vi "AlliGator Load ROI v3.vi"(7 "File Path":path, 8 "Error In":errorcluster, 9 "Destination Image (Source Image)":string="Source Image", 10 "Dialog (T)":bool=TRUE, 11 "Source Image Refnum":T3) -> (0 "Error Out":errorcluster, 1 "Current ROI":i32, 2 "Updated ROIs":T1[](array[typedef]) {"ROI Descriptor"."Contours"."Type" items=["No Selection", "Point", "Line", "Rectangle", "Oval", "Polygon", "Freehand Region", "Annulus", "Unused2", "Unused3", "Broken Line", "Freehand Line", "Rotated Rectangle"]}, 3 "Message":string, 4 "Phasor Plot Image":bool, 5 "# ROIs Loaded":i32, 6 "Time (s)":dbl)   [LabVIEW 2021, in "AlliGator ROIs.lvlib"]
doc: "When invoked from a context menu, used Dialog for file selection: the Dialog flag should be set to True (default) and the Destination Image string is ignored.\n\nWhen invoked from a drag & drop event, the Dialog flag should be set to False and the Destination Image (Source Image or Phasor Plot Image) should be provided."
uses:
  AlliGator ROIs.lvlib
  Image/Image Control Refnum.ctl
  Image/Named ROI Description.ctl
  Globals, Variables, Constants/AlliGator Refnums List.ctl
  Globals, Variables, Constants/AlliGator Variables List.ctl
  Image/ROI XML Format.ctl
  Image/Image Control ROI Description.ctl
  Image/Image Control Multiple ROIs Description.ctl
  Image/Image Control ROI Description v2.ctl
  Image/Image Control Multiple ROIs Description v2.ctl
  AlliGator ROI Manager Actions.ctl
  8ad5fe3a-6877-4cbc-8fef-4c072b65eab6.vi
  454e6171-cdfd-4cb8-a5e3-eaa046060a80.vi
  Variant/Variant to Data/Variant to I32.vi
  <vilib>/JDP Science/JSONtext/JSON text to Variant.vi
  <vilib>/Utility/error.llb/Error Cluster From Error Code.vi
  <vilib>/JDP Science/JSONtext/LVClass Serializer/JSONtext LVClass Serializer.lvclass
  <vilib>/ErrorRing/Error Ring.xnode
  Image/Image.lvlib
  Files/Files.lvlib
  Error/Error.lvlib
  Globals, Variables, Constants/AlliGator Globals, Variables & Constants.lvlib
  Variant/Variant to Data/Variant to Data.lvlib
  Time/Time.lvlib
  Sound/Sound.lvlib
panel:
  # "see the AlliGator License on the block diagram (Ctrl+E or Window:Show Block Diagram)"
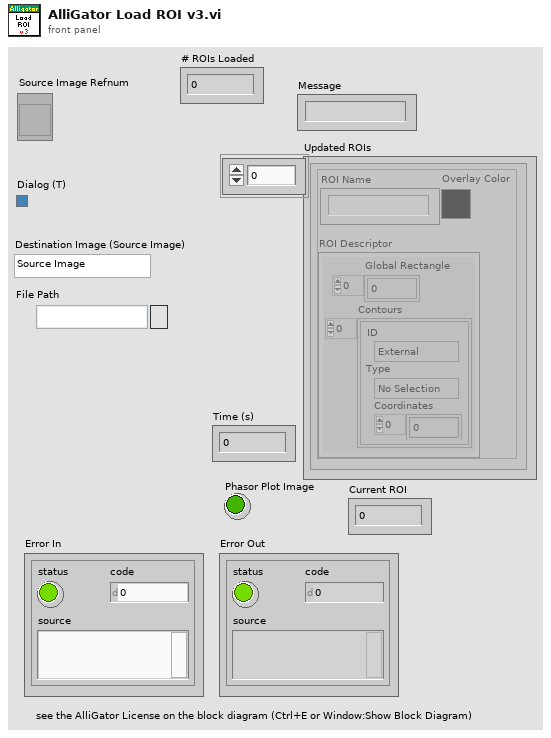
[diagram p1: front panel]
types:
  T1 = typedef "Image.lvlib/Named ROI Description.ctl" = cluster{"ROI Descriptor":T2, "ROI Name":string, "Overlay Color":u32}
  T2 = typedef "ROI Descriptor" = cluster{"Global Rectangle":i32[], "Contours":cluster{"ID":enum32{"External", "Internal"}, "Type":u32, "Coordinates":i32[]}[]}
  T3 = typedef "Image.lvlib/Image Control Refnum.ctl" = refnum<vi>
  T4 = typedef "AlliGator Globals, Variables & Constants.lvlib/AlliGator Refnums List.ctl" = enum16{"---------- AlliGator Controls ----------", "AlliGator Tab Control Refnum", "---------- AlliGator Indicators ----------", "Source Image Display Refnum", "Phasor Plot Display Refnum", "Decay Fit Parameter Map Refnum", "---------- AlliGator VIs ----------", "AlliGator Refnum", "AlliGator Settings Refnum", "AlliGator Launcher Refnum"}
  T5 = typedef "AlliGator Globals, Variables & Constants.lvlib/AlliGator Variables List.ctl" = enum16{"---- GUI ----", "GUI:Initialization Status", "GUI:State Indicators Refnum", "GUI:Original AlliGator Menu Items", "GUI:Current Action Loop State", "GUI:Script in progress", "GUI:Playback", "GUI:Loop Playback", "GUI:Search ROI Used", "GUI:Search ROI", "Decay Graph Max Legend Size", "Intensity Graph Max Legend Size", "Decay Statistics Graph Max Legend Size", "Phasor Graph Max Legend Size", "Phasor Ratio Graph Max Legend Size", "Lifetime Graph Max Legend Size", "---- Files ----", "Files:Export Dataset Frames as Individual Files", "Files:Show Batch Export Help Balloons", "Files:Frames in Dataset", "Files:ptu File Frame Start Indices", "Files:Current Frame in Dataset", "Files:Current Frame Timestamp", "Files:Dataset Loaded", "Files:Dataset Metadata", "Files:Dataset Channel", "Files:Dataset Data Description", "Files:Background Dataset Metadata", "Files:Background Dataset Channel", "Files:Background Dataset Data Description", "Files:Background File Subtraction", "Files:Background File Path", "Files:Background File Pile-up Correction", "Files:Background File Pixel Well Capacity", "Files:Background File Scaling Factor", "Files:Current Dataset Load Settings", "Files:Dataset Path", "Files:ICCD-specific Information", "Files:Macrotime Gate Separation", "------ Python Plugins ------", "Python Plugins:Information", "Python Plugins:Python Session", "Python Plugins:Valid Python Session?", "---- Source Image ----", "Source Image:ROIs", "Source Image:Current ROI", "Source Image:ROI Event Refnum", "X_Source Image:Display Range", "X_Source Image:Palette Information", "X_Source Image:Type of Displayed Image", "X_Time Gate Slider", "Source Image:Palette List", "Source Image:Scale", "Source Image:ROI Overlay Color", "Source Image:Overlay to Erase", "Source Image:Is Displayed Image Accumulated", "Source Image:White Light Image Modified", "Source Image:Mask Image Modified", "---- Image Profile Window ----", "Image Profile:Window Event Refnum", "Image Profile:IntensityType", "Image Profile:Intensity Average Type", "Image Profile:Intensity-weighted SDV", "Image Profile:Box Profile Type", "Image Profile:Window Open", "Image Profile:Plotted Fit Parameter", "------ Phasor Graph -------", "Phasor Graph:Show Line", "---- Phasor Plot ---", "Phasor Plot:Parameters Changed", "Phasor Plot:FLI Dataset Modified since last Calculation", "Phasor Harmonics Data", "Selected Phasor Harmonics", "Phasor Harmonic Manager Event Refnum", "Phasor Plot:ROIs", "Phasor Plot:Current ROI", "Phasor Plot:ROI Event Refnum", "Phasor Plot:Image Reference Points", "Phasor Plot:Computed", "Phasor Plot:Palette Information", "Phasor Plot:Palette List", "Phasor Plot:Phasor Ratio Palette Information", "Phasor Plot:Phasor Ratio Palette List", "Phasor Plot:Image Scale", "Phasor Plot:Image Overlay to Erase", "Phasor Plot:Image Elements to Update", "Phasor Plot:Current Calculation Parameters", "Phasor Plot:Current Calibration Options", "Phasor Plot:Reset Cumulated Phasor Plot", "Phasor Plot:Reference 1", "Phasor Plot:Lifetime Reference 1", "Phasor Plot:Reference 1 Frequency", "Phasor Plot:Reference 2", "Phasor Plot:Lifetime Reference 2", "Phasor Plot:Reference 2 Frequency", "---- Decay Analysis ----", "Number of Selected Decays to Fit", "LS Fit Results", "LAR Fit Results", "BS Fit Results", "Last Decay Max - Min", "Best Fit Parameters", "Best Fit Parameter Names", "Actual Size X", "Actual Size Y", "Binning X", "Binning Y", "Actual # Gates", "Dataset Number", "Gates to...", "Gates Skipped", "Gates to keep", "Gate Step", "Gate Separation", "Reversed Gates", "Pile-up Correction", "Pixel Well Capacity", "Background Subtracted", "Background Subtraction Method", "Background Definition Range", "Background File (deprecated)", "Number of Dataset Accumulated", "Array of Accumulated Dataset Paths", "Do Averaged Datasets", "Destination File Path", "Process Plot Target", "Use 1/D as Phasor Frequency", "---- Decay Fit Parameter Map -----", "Decay Fit Parameter Map:Palette Information", "Decay Fit Parameter Map:Palette List", "Decay Fit Parameter Map:X Resolution", "Decay Fit Parameter Map:Y Resolution", "---- Parameter Map ----", "Parameter Map:Palette Information", "Parameter Map:Palette List", "------- Local Decay Window ---------", "Local Decay Graph Window:Event Refnum", "Local Decay Graph Window:Use normalized IRF for convolution", "----- Miscellaneous ----", "Misc:Skippable Dialog Windows Status"}
  T6 = typedef "Image.lvlib/ROI XML Format.ctl" = enum16{"Single ROI v1", "Multiple ROIs v1", "Single ROI v2", "Multiple ROIs v2", "Single ROI v3", "Multiple ROIs v3", "Exit"}
  T7 = typedef "Image.lvlib/Image Control ROI Description.ctl" = cluster{"Image Control Label":string, "ROI Descriptor":T2}
  T8 = typedef "Image.lvlib/Image Control Multiple ROIs Description.ctl" = cluster{"Image Control Label":string, "ROI Descriptors":T2[]}
  T9 = typedef "Image.lvlib/Image Control ROI Description v2.ctl" = cluster{"Image Control Label":string, "Named ROI Description":T1}
  T10 = typedef "Image.lvlib/Image Control Multiple ROIs Description v2.ctl" = cluster{"Image Control Label":string, "Named ROI Descriptions":T1[]}
  T11 = typedef "AlliGator ROIs.lvlib/AlliGator ROI Manager Actions.ctl" = enum16{"Undefined", "Delete Current ROI", "Delete All Unselected ROIs", "Delete Multiple ROIs", "Delete All ROIs", "Swap ROIs", "Insert ROI", "Update Current ROI Descriptor", "Rename Current ROI", "Store New ROI", "Store Multiple ROIs", "Select Next ROI", "Select Previous ROI", "Find Selected ROI", "Show All ROIs", "Update ROI Manager Window", "Merge All ROIs", "Unmerge ROI", "Set Selected ROI by ID"}
  T12 = typedef "AlliGator ROIs.lvlib/AlliGator Image ROI Event refnum.ctl" = refnum<user-event>
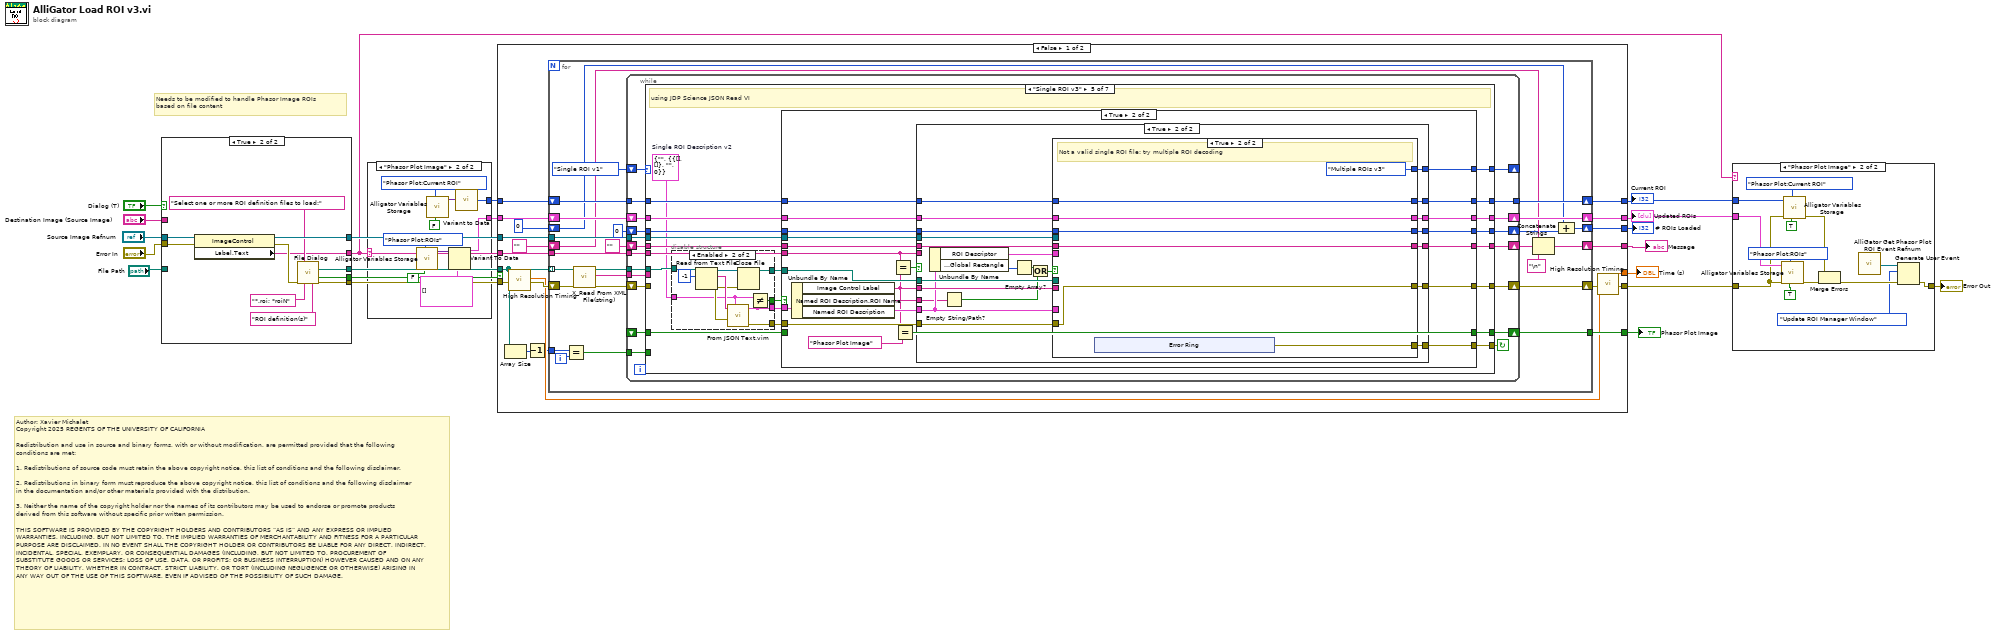
[diagram p0: block diagram]
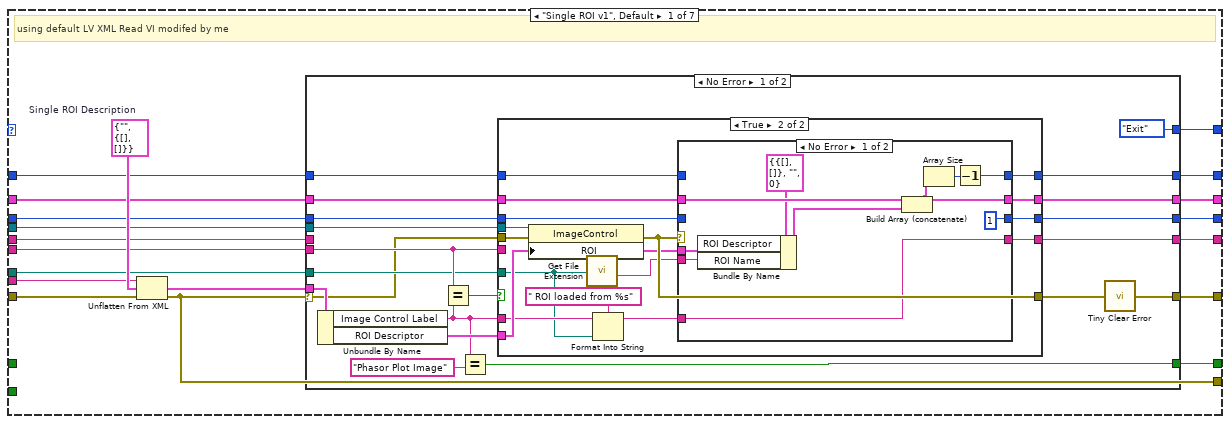
[diagram p2: hidden frame]
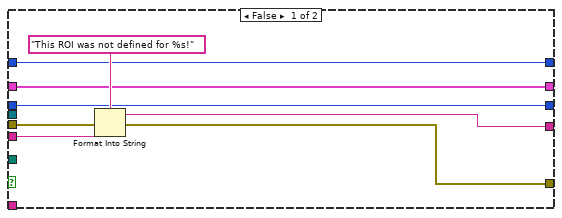
[diagram p3: hidden frame]
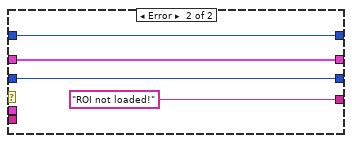
[diagram p4: hidden frame]
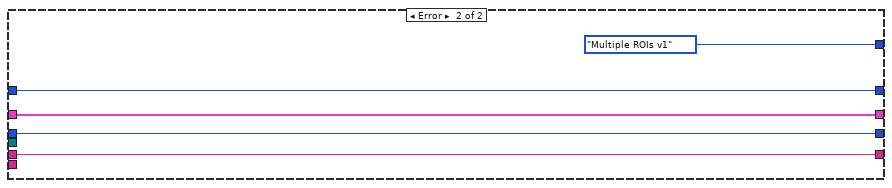
[diagram p5: hidden frame]
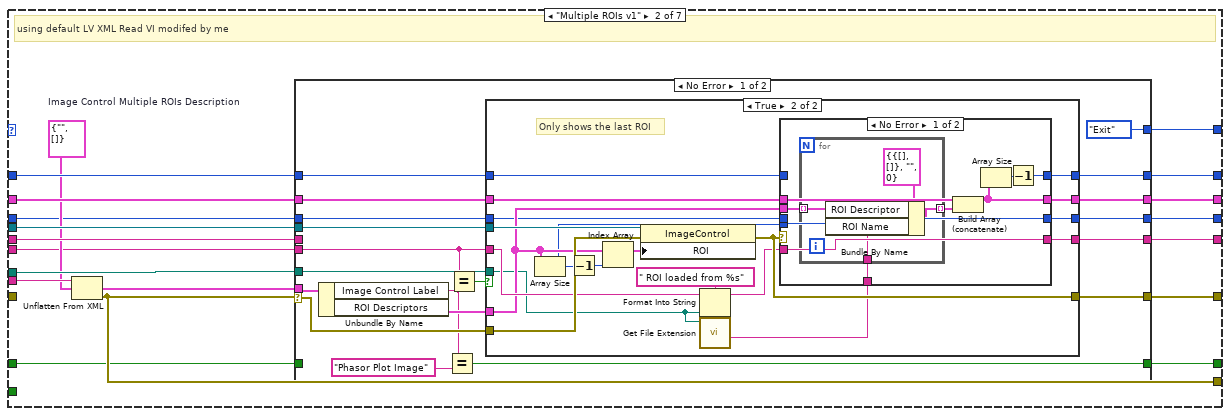
[diagram p6: hidden frame]
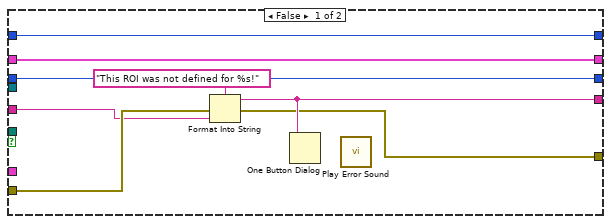
[diagram p7: hidden frame]
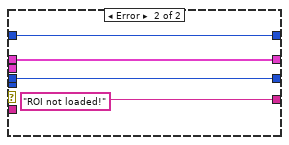
[diagram p8: hidden frame]
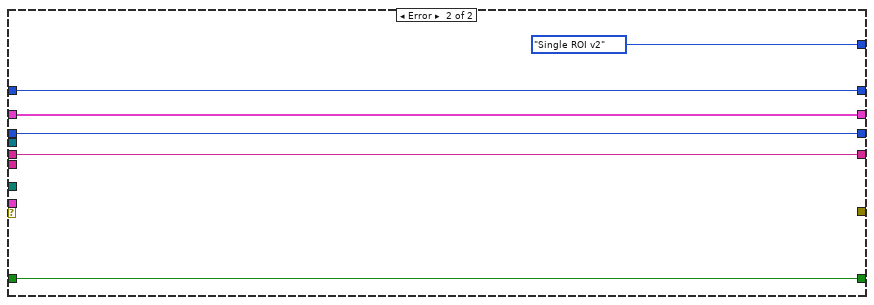
[diagram p9: hidden frame]
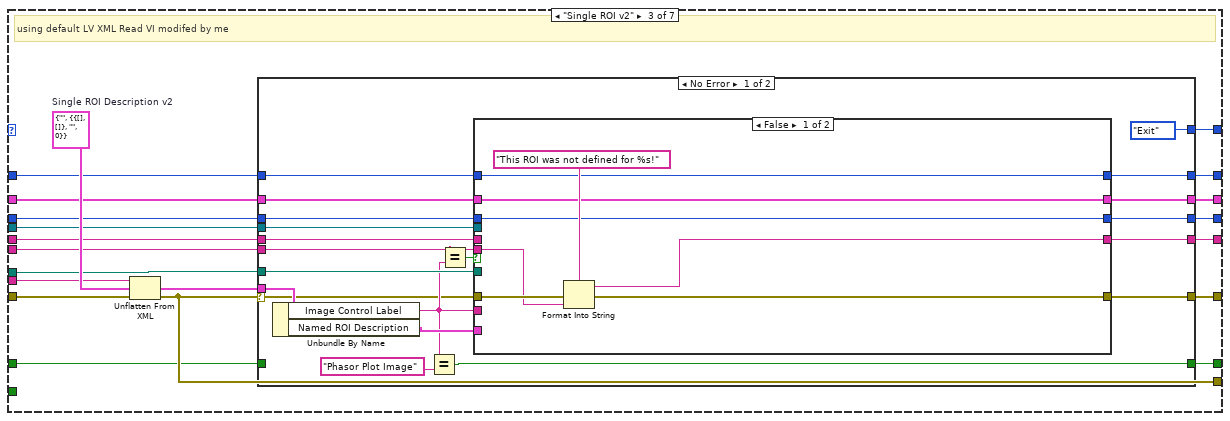
[diagram p10: hidden frame]
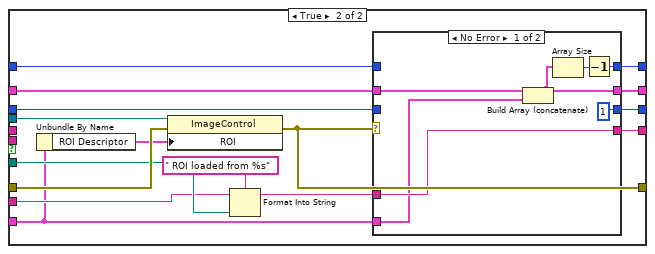
[diagram p11: hidden frame]
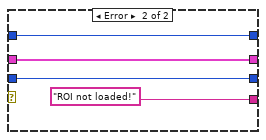
[diagram p12: hidden frame]
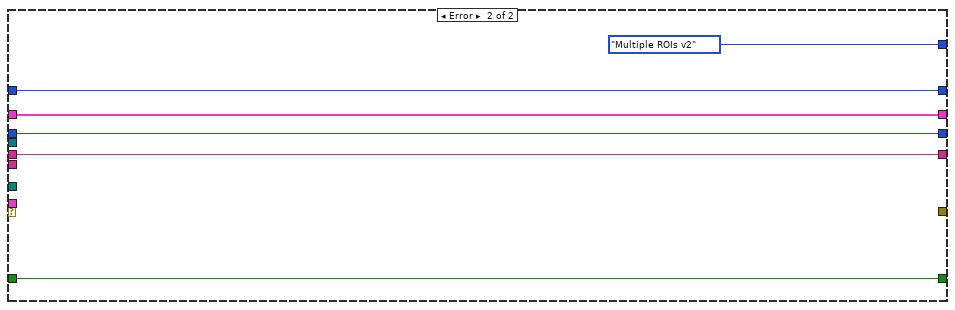
[diagram p13: hidden frame]
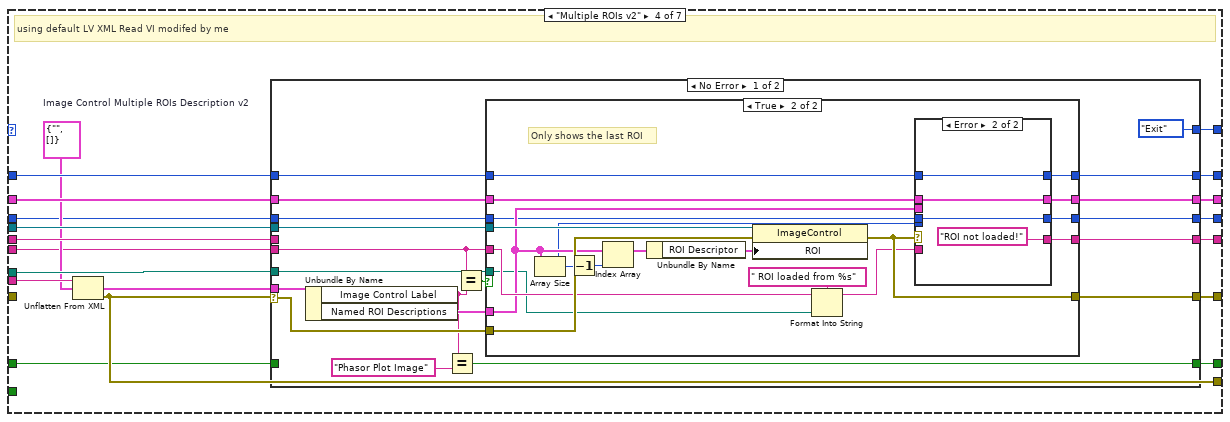
[diagram p14: hidden frame]
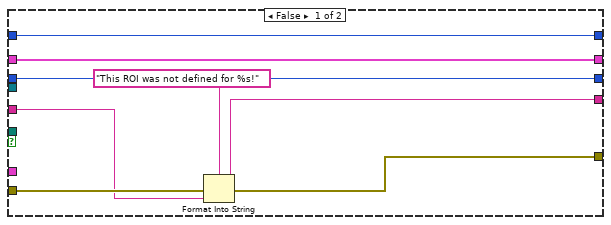
[diagram p15: hidden frame]
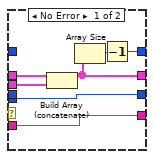
[diagram p16: hidden frame]
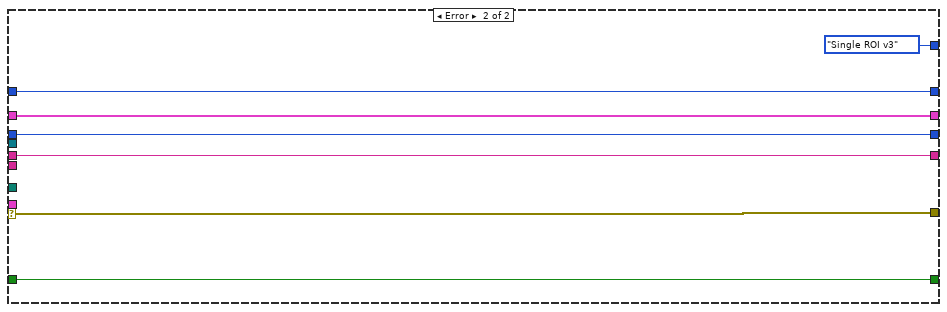
[diagram p17: hidden frame]
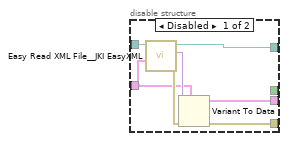
[diagram p18: hidden frame]
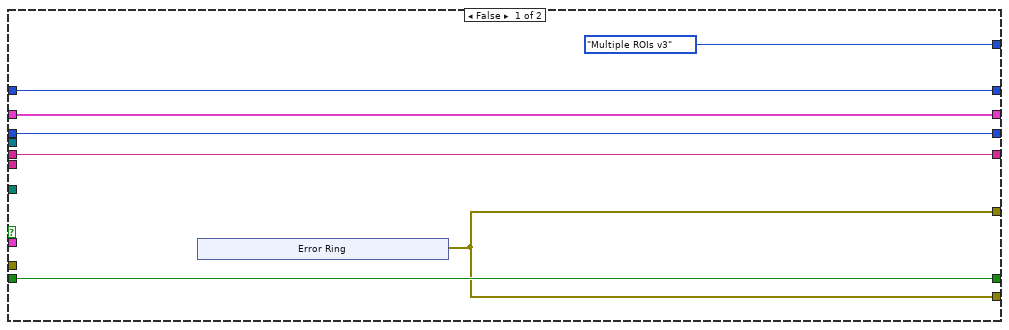
[diagram p19: hidden frame]
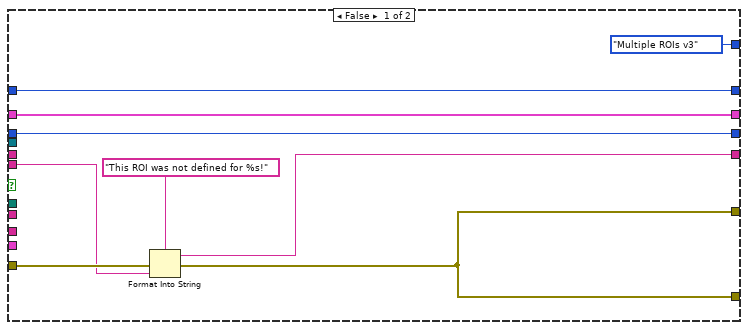
[diagram p20: hidden frame]
diagram:
  # "Author: Xavier Michalet\nCopyright 2025 REGENTS OF THE UNIVERSITY OF CALIFORNIA\n\nRedistribution and use in source and binary forms, with or without modification, are permitted provided that the following conditions are met:\n\n1. Redistributions of source code must retain the above copyright notice, this list of conditions and the following disclaimer.\n\n2. Redistributions in binary form must reproduce the above copyright notice, this list of conditions and the following disclaimer in the documentation and/or other materials provided with the distribution.\n\n3. Neither the name of the copyright holder nor the names of its contributors may be used to endorse or promote products derived from this software without specific prior written permission.\n\nTHIS SOFTWARE IS PROVIDED BY THE COPYRIGHT HOLDERS AND CONTRIBUTORS “AS IS” AND ANY EXPRESS OR IMPLIED WARRANTIES, INCLUDING, BUT NOT LIMITED TO, THE IMPLIED WARRANTIES OF MERCHANTABILITY AND FITNESS FOR A PARTICULAR PURPOSE ARE DISCLAIMED. IN NO EVENT SHALL THE COPYRIGHT HOLDER OR CONTRIBUTORS BE LIABLE FOR ANY DIRECT, INDIRECT, INCIDENTAL, SPECIAL, EXEMPLARY, OR CONSEQUENTIAL DAMAGES (INCLUDING, BUT NOT LIMITED TO, PROCUREMENT OF SUBSTITUTE GOODS OR SERVICES; LOSS OF USE, DATA, OR PROFITS; OR BUSINESS INTERRUPTION) HOWEVER CAUSED AND ON ANY THEORY OF LIABILITY, WHETHER IN CONTRACT, STRICT LIABILITY, OR TORT (INCLUDING NEGLIGENCE OR OTHERWISE) ARISING IN ANY WAY OUT OF THE USE OF THIS SOFTWARE, EVEN IF ADVISED OF THE POSSIBILITY OF SUCH DAMAGE."
  # "Needs to be modified to handle Phasor Image ROIs\nbased on file content"
  n1 = case shown="True" "Dialog (T)" {
    tunnel: "Source Image Refnum" -> [_ w46]
    tunnel: [w22 w45] -> w19
    tunnel: "Error In" -> [w21 w44]
    tunnel: [w21 w42] -> w16
    tunnel: [w24 w38] -> w15
    tunnel: [_ w37] -> w13
    tunnel: [w23 w36] -> w8
    tunnel: "Destination Image (Source Image)" -> [w23 _]
    tunnel: "File Path" -> [w25 _]
    frame False {
      # "Drag & Drop event"
      n2 = case shown="\"Phasor Plot Image\"" w23 {
        tunnel: [w27 w32] -> w22
        frame "Source Image", Default {
          n3 = call "AlliGator Refnums Storage.vi"("AlliGator Refnum List"=AlliGator_Refnums_List."Source Image Display Refnum") -> ("Error Out"=w29:errorcluster, "Data out"=w30:variant)  [unwired: 9 in]
          n4 = Variant To Data(error in=w29, type=refnum<vi> refnum ("Image Source Refnum"), Variant=w30) -> (data=w27:refnum<vi>)  [unwired: 1 out]
        }
        frame "Phasor Plot Image" {
          n5 = call "AlliGator Refnums Storage.vi"("AlliGator Refnum List"=AlliGator_Refnums_List."Phasor Plot Display Refnum") -> ("Error Out"=w34:errorcluster, "Data out"=w35:variant)  [unwired: 9 in]
          n6 = Variant To Data(error in=w34, type=refnum<vi> refnum ("Image Source Refnum"), Variant=w35) -> (data=w32:refnum<vi>)  [unwired: 1 out]
        }
      }
      n7 = Build Array(w25) -> (w24:path[])
    }
    frame True {
      n8 = property class="ImageControl"(reference=w46, error in=w44) -> (reference out=w45:T3, error out=w43:errorcluster, "Label.Text"=w36:string)
      n9 = call "File Dialog"("prompt"="Select one or more ROI definition files to load:", "error in"=w43, "pattern (all files)"="*.roi; *roiN", "pattern label"="ROI definition(s)") -> ("selected paths"=w38:path[], "cancelled"=w37:bool, "error out"=w42:errorcluster)  [unwired: 8 in, 1 out]
    }
  }
  n10 = case shown="\"Phasor Plot Image\"" w8 {
    tunnel: [w53 w63] -> w12
    tunnel: [w47 w57] -> w11
    frame "Source Image", Default {
      n11 = call "Alligator Variables Storage.vi"("Get(F)/Set"=FALSE, "AlliGator Variable"=AlliGator_Variables_List."Source Image:ROIs" ("Alligator Variable")) -> ("Error Out"=w49:errorcluster, "Data out"=w50:variant)  [unwired: 7 in, 1 out]
      n12 = call "Alligator Variables Storage.vi"("Get(F)/Set"=FALSE, "AlliGator Variable"=AlliGator_Variables_List."Source Image:Current ROI" ("Alligator Variable")) -> ("Data out"=w54:variant)  [unwired: 7 in, 2 out]
      n13 = Variant To Data(error in=w49, type=T1[] [] ("Existing ROIs"), Variant=w50) -> (data=w47:T1[])  [unwired: 1 out]
      n14 = call-poly "Variant to Data.vi"("Variant"=w54) -> ("Value"=w53:i32)  [unwired: 8 in]
    }
    frame "Phasor Plot Image" {
      n15 = call "Alligator Variables Storage.vi"("Get(F)/Set"=FALSE, "AlliGator Variable"=AlliGator_Variables_List."Phasor Plot:ROIs" ("Alligator Variable")) -> ("Error Out"=w59:errorcluster, "Data out"=w60:variant)  [unwired: 7 in, 1 out]
      n16 = call "Alligator Variables Storage.vi"("Get(F)/Set"=FALSE, "AlliGator Variable"=AlliGator_Variables_List."Phasor Plot:Current ROI" ("Alligator Variable")) -> ("Data out"=w64:variant)  [unwired: 7 in, 2 out]
      n17 = Variant To Data(error in=w59, type=T1[] [] ("Existing ROIs"), Variant=w60) -> (data=w57:T1[])  [unwired: 1 out]
      n18 = call-poly "Variant to Data.vi"("Variant"=w64) -> ("Value"=w63:i32)  [unwired: 8 in]
    }
  }
  n19 = case shown="False" w13 {
    tunnel: w8 -> [w86 _]
    tunnel: w19 -> [w85 _]
    tunnel: w11 -> [w84 w728]
    tunnel: [w83 w728] -> w9
    tunnel: [w72 w729] -> w1
    tunnel: w12 -> [w81 _]
    tunnel: [w80 -1 ("Current ROI")] -> w10
    tunnel: [w79 _] -> w17
    tunnel: w16 -> [w78 w729]
    tunnel: w15 -> [w69 _]
    tunnel: [w77 "ROI Loading cancelled by user..."] -> w2
    tunnel: [w74 _] -> w14
    tunnel: [w70 _] -> w6
    frame False {
      n20 = Array Size(array=w69) -> (size(s)=w68:i32)
      n21 = call "High Resolution Timing.vi"("Error In"=w78) -> ("elapsed (relative) seconds"=w71:dbl, "Error Out"=w73:errorcluster)  [unwired: 16 in, 1 out]
      n22 = Decrement(x=w68) -> (x-1=w67:i32)
      n23 = for {
        tunnel: w85 -> [w111]
        tunnel: [w104] -> w79
        shift-right: [w105] -> w80
        shift-left: w81 -> [w106]
        shift-right: [w89] -> w82
        shift-left: w73 -> [w103]
        shift-right: [w107] -> w83
        shift-left: w84 -> [w108]
        tunnel: w69 -> [w102] mode=indexing
        tunnel: w86 -> [w87]
        shift-right: [w99] -> w77
        shift-left: "" -> [w98]
        shift-right: [w97] -> w74
        shift-left: 0 -> [w96]
        tunnel: w67 -> [w92]
        i -> [w91]
        n24 = Equal?(x=w92, y=w91) -> (x = y?=w90:bool)
        n25 = call "X_Read From XML File(string).vi"("error in (no error)"=w103, "XML File Path"=w102) -> ("error out"=w112:errorcluster, "XML Elements"=w109:string, "XML File Path(duplicate)"=w110:path)  [unwired: 7 in]
        n26 = while {
          tunnel: w111 -> [w130]
          tunnel: w110 -> [w129]
          tunnel: w109 -> [w128]
          tunnel: w106 -> [w125]
          tunnel: [w124] -> w105
          shift-right: [w119] -> w89
          shift-left: w112 -> [w132]
          shift-right: [w122] -> w100
          shift-left: "" -> [w131]
          shift-right: [w126] -> w107
          shift-left: w108 -> [w127]
          shift-right: [w117] -> _
          shift-left: ROI_XML_Format."Single ROI v1" -> [w120]
          shift-right: [w121] -> w95
          shift-left: 0 ("value") -> [w116]
          tunnel: w90 -> [w115]
          shift-right: [w123] -> w104
          shift-left: _ -> [w114]
          tunnel: w87 -> [w113]
          stop <- w118 continue-if-true
          n27 = case shown="\"Single ROI v3\"" w120 {
            selector: w120 -> [_ _ _ _ _ _ w724]
            tunnel: w132 -> [w150 _ w321 _ _ _ w718]
            tunnel: w131 -> [w133 w233 w319 w402 w470 w627 w721]
            tunnel: w130 -> [w148 w232 w318 w401 w487 w626 _]
            tunnel: w129 -> [w147 w231 w317 w400 w477 w617 _]
            tunnel: w128 -> [w146 w230 w316 w399 _ _ _]
            tunnel: w127 -> [w145 w229 w315 w398 w486 w625 w722]
            tunnel: [w144 w228 w314 w397 w485 w624 w722] -> w126
            tunnel: [w136 w219 w306 w388 w478 w608 w719] -> w119
            tunnel: w125 -> [w143 w227 w313 w396 w484 w623 w723]
            tunnel: [w142 w226 w312 w395 w483 w622 w723] -> w124
            tunnel: [w141 w218 w311 w387 w482 w618 w716] -> w123
            tunnel: [w140 w225 w310 w394 w481 w621 w721] -> w122
            tunnel: [w139 w224 w309 w393 w480 w620 _] -> w121
            tunnel: [w138 w221 w308 w390 w469 w608 w717] -> w118
            tunnel: [w137 w220 w307 w389 w479 w619 w724] -> w117
            tunnel: w116 -> [w135 w217 w305 w386 w473 w613 _]
            tunnel: w115 -> [_ _ _ _ _ _ w720]
            tunnel: w114 -> [_ w216 w304 w385 w472 w612 w716]
            tunnel: w113 -> [w134 w215 w303 w384 w471 w611 _]
            frame "Single ROI v1", Default {
              w151 = T7 {"Image Control Label"="", "ROI Descriptor"={"Global Rectangle"=[], "Contours"=[]}}  # Single ROI Description
              # "using default LV XML Read VI modifed by me"
              n28 = Unflatten From XML(xml string=w146, type=w151, error in (no error)=w150) -> (value=w149:T7, error out=w138:errorcluster)
              n29 = case shown="No Error" w138 {
                selector: w138 -> [w157 _]
                tunnel: w149 -> [w171 _]
                tunnel: w134 -> [w170 _]
                tunnel: w148 -> [w169 _]
                tunnel: w147 -> [w168 _]
                tunnel: w145 -> [w167 w214]
                tunnel: [w166 w214] -> w144
                tunnel: [w155 _] -> w136
                tunnel: w143 -> [w164 w213]
                tunnel: [w163 w213] -> w142
                tunnel: [w152 _] -> w141
                tunnel: [w162 w210] -> w140
                tunnel: [w161 w211] -> w139
                tunnel: [ROI_XML_Format."Exit" ROI_XML_Format."Multiple ROIs v1"] -> w137
                tunnel: w135 -> [w154 w211]
                tunnel: w133 -> [_ w210]
                frame No Error {
                  n30 = Unbundle By Name(w171) -> ("Image Control Label"=w158:string, "ROI Descriptor"=w159:T2)
                  n31 = Equal?(x=w170, y=w158) -> (x = y?=w160:bool)
                  n32 = Equal?(x=w158, y="Phasor Plot Image") -> (x = y?=w152:bool)
                  n33 = case shown="True" w160 {
                    tunnel: w159 -> [_ w190]
                    tunnel: w169 -> [_ w195]
                    tunnel: w157 -> [w175 w194]
                    tunnel: [w177 w188] -> w162
                    tunnel: w168 -> [_ w182]
                    tunnel: w158 -> [_ w184]
                    tunnel: w170 -> [w178 _]
                    tunnel: w167 -> [w176 w191]
                    tunnel: [w176 w189] -> w166
                    tunnel: [w174 w192] -> w165
                    tunnel: w164 -> [w173 w186]
                    tunnel: [w173 w185] -> w163
                    tunnel: [w172 w183] -> w161
                    tunnel: w154 -> [w172 w180]
                    frame False {
                      n34 = Format Into String(format string="This ROI was not defined for %s!" ("message"), error in=w175, w178) -> (resulting string=w177:string, error out=w174:errorcluster)  [unwired: 1 in]
                    }
                    frame True {
                      n35 = property class="ImageControl"(reference=w195, error in=w194, "ROI"=w190) -> (error out=w192:errorcluster)  [unwired: 1 out]
                      n36 = call <vilib>:"Get File Extension.vi"("file"=w182) -> ("filename without extension"=w181:string)  [unwired: 6 in, 4 out]
                      n37 = Format Into String(format string=" ROI loaded from %s", initial string=w184, w182) -> (resulting string=w187:string)  [unwired: 1 in, 1 out]
                      n38 = case shown="No Error" w192 {
                        tunnel: w191 -> [w205 w209]
                        tunnel: w190 -> [w198 _]
                        tunnel: [w203 w209] -> w189
                        tunnel: [w204 "ROI not loaded!" ("t")] -> w188
                        tunnel: w187 -> [w204 _]
                        tunnel: w186 -> [_ w207]
                        tunnel: [w201 w207] -> w185
                        tunnel: [1 ("value") w206] -> w183
                        tunnel: w181 -> [w197 _]
                        tunnel: w180 -> [_ w206]
                        frame No Error {
                          n39 = Bundle By Name(cluster=T1 {"ROI Descriptor"={"Global Rectangle"=[], "Contours"=[]}, "ROI Name"="", "Overlay Color"=0} ("Named ROI Description"), "ROI Descriptor"=w198, "ROI Name"=w197) -> (w196:T1)
                          n40 = Build Array (concatenate)(w205, w196) -> (w203:T1[])
                          n41 = Array Size(array=w203) -> (size(s)=w202:i32)
                          n42 = Decrement(x=w202) -> (x-1=w201:i32)
                        }
                        frame Error {
                        }
                      }
                    }
                  }
                  n43 = call "Tiny Clear Error.vi"("Error In"=w165) -> ("no Error Out"=w155:errorcluster)  [unwired: 8 in]
                }
                frame Error {
                }
              }
            }
            frame "Multiple ROIs v1" {
              w223 = T8 {"Image Control Label"="", "ROI Descriptors"=[]}  # Image Control Multiple ROIs Description
              # "using default LV XML Read VI modifed by me"
              n44 = Unflatten From XML(xml string=w230, type=w223) -> (value=w222:T8, error out=w221:errorcluster)  [unwired: 1 in]
              n45 = case shown="No Error" w221 {
                selector: w221 -> [w245 _]
                tunnel: w222 -> [w252 _]
                tunnel: w233 -> [_ w300]
                tunnel: w229 -> [w250 w302]
                tunnel: [w249 w302] -> w228
                tunnel: [w248 _] -> w219
                tunnel: w231 -> [w247 _]
                tunnel: w232 -> [w246 _]
                tunnel: w227 -> [w243 w301]
                tunnel: [w242 w301] -> w226
                tunnel: [w241 w300] -> w225
                tunnel: [w240 w298] -> w224
                tunnel: [ROI_XML_Format."Exit" ROI_XML_Format."Single ROI v2"] -> w220
                tunnel: [w236 w297] -> w218
                tunnel: w217 -> [w235 w298]
                tunnel: w216 -> [_ w297]
                tunnel: w215 -> [w234 _]
                frame No Error {
                  n46 = Unbundle By Name(w252) -> ("Image Control Label"=w237:string, "ROI Descriptors"=w244:T2[])
                  n47 = Equal?(x=w237, y="Phasor Plot Image") -> (x = y?=w236:bool)
                  n48 = Equal?(x=w234, y=w237) -> (x = y?=w251:bool)
                  n49 = case shown="True" w251 {
                    tunnel: w246 -> [_ w279]
                    tunnel: w245 -> [w257 w278]
                    tunnel: [w259 w272] -> w241
                    tunnel: w247 -> [_ w263]
                    tunnel: w234 -> [w255 w277]
                    tunnel: w250 -> [w258 w274]
                    tunnel: [w258 w273] -> w249
                    tunnel: [w256 w275] -> w248
                    tunnel: w244 -> [_ w269]
                    tunnel: w243 -> [w254 w267]
                    tunnel: [w254 w266] -> w242
                    tunnel: [w253 w264] -> w240
                    tunnel: w235 -> [w253 w261]
                    frame False {
                      n50 = Format Into String(format string="This ROI was not defined for %s!" ("message"), error in=w257, w255) -> (resulting string=w259:string, error out=w256:errorcluster)  [unwired: 1 in]
                      n51 = One Button Dialog(message=w259) -> ()  [unwired: 1 in, 1 out]
                      n52 = call "Play Error Sound.vi"() -> ()  [unwired: 27 in, 1 out]
                    }
                    frame True {
                      # "Only shows the last ROI"
                      n53 = Array Size(array=w269) -> (size(s)=w265:i32)
                      n54 = Decrement(x=w265) -> (x-1=w268:i32)
                      n55 = Index Array(array=w269, index=w268) -> (element=w270:T2)
                      n56 = property class="ImageControl"(reference=w279, error in=w278, "ROI"=w270) -> (error out=w275:errorcluster)  [unwired: 1 out]
                      n57 = Format Into String(format string=" ROI loaded from %s", initial string=w277, w263) -> (resulting string=w271:string)  [unwired: 1 in, 1 out]
                      n58 = call <vilib>:"Get File Extension.vi"("file"=w263) -> ("filename without extension"=w262:string)  [unwired: 6 in, 4 out]
                      n59 = case shown="No Error" w275 {
                        tunnel: w274 -> [w288 w296]
                        tunnel: [w286 w296] -> w273
                        tunnel: [w287 "ROI not loaded!" ("t")] -> w272
                        tunnel: w271 -> [w287 _]
                        tunnel: w269 -> [w282 _]
                        tunnel: w267 -> [_ w294]
                        tunnel: [w284 w294] -> w266
                        tunnel: w265 -> [w283 _]
                        tunnel: [w283 w293] -> w264
                        tunnel: w262 -> [w280 _]
                        tunnel: w261 -> [_ w293]
                        frame No Error {
                          n60 = for {
                            tunnel: w282 -> [w292] mode=indexing
                            tunnel: [w290] -> w281 mode=indexing
                            tunnel: w280 -> [w289]
                            n61 = Bundle By Name(cluster=T1 {"ROI Descriptor"={"Global Rectangle"=[], "Contours"=[]}, "ROI Name"="", "Overlay Color"=0} ("Named ROI Description"), "ROI Descriptor"=w292, "ROI Name"=w289) -> (w290:T1)
                          }
                          n62 = Build Array (concatenate)(w288, w281) -> (w286:T1[])
                          n63 = Array Size(array=w286) -> (size(s)=w285:i32)
                          n64 = Decrement(x=w285) -> (x-1=w284:i32)
                        }
                        frame Error {
                        }
                      }
                    }
                  }
                }
                frame Error {
                }
              }
            }
            frame "Single ROI v2" {
              w322 = T9 {"Image Control Label"="", "Named ROI Description"={"ROI Descriptor"={"Global Rectangle"=[], "Contours"=[]}, "ROI Name"="", "Overlay Color"=0}}  # Single ROI Description v2
              # "using default LV XML Read VI modifed by me"
              n65 = Unflatten From XML(xml string=w316, type=w322, error in (no error)=w321) -> (value=w320:T9, error out=w308:errorcluster)
              n66 = case shown="No Error" w308 {
                selector: w308 -> [w328 _]
                tunnel: w320 -> [w342 _]
                tunnel: w319 -> [w341 w383]
                tunnel: w318 -> [w340 _]
                tunnel: w317 -> [w339 _]
                tunnel: w315 -> [w338 w382]
                tunnel: [w337 w382] -> w314
                tunnel: [w336 _] -> w306
                tunnel: w313 -> [w335 w381]
                tunnel: [w334 w381] -> w312
                tunnel: [w323 w378] -> w311
                tunnel: [w333 w383] -> w310
                tunnel: [w332 w379] -> w309
                tunnel: [ROI_XML_Format."Exit" ROI_XML_Format."Multiple ROIs v2"] -> w307
                tunnel: w305 -> [w326 w379]
                tunnel: w304 -> [_ w378]
                tunnel: w303 -> [w325 _]
                frame No Error {
                  n67 = Unbundle By Name(w342) -> ("Image Control Label"=w329:string, "Named ROI Description"=w330:T1)
                  n68 = Equal?(x=w329, y="Phasor Plot Image") -> (x = y?=w323:bool)
                  n69 = Equal?(x=w325, y=w329) -> (x = y?=w331:bool)
                  n70 = case shown="False" w331 {
                    tunnel: w330 -> [_ w352]
                    tunnel: w340 -> [_ w366]
                    tunnel: w328 -> [w347 w365]
                    tunnel: [w349 w359] -> w333
                    tunnel: w339 -> [_ w363]
                    tunnel: w329 -> [_ w355]
                    tunnel: w341 -> [_ _]
                    tunnel: w338 -> [w348 w361]
                    tunnel: [w348 w360] -> w337
                    tunnel: [w346 w362] -> w336
                    tunnel: w335 -> [w345 w357]
                    tunnel: [w345 w356] -> w334
                    tunnel: [w344 w354] -> w332
                    tunnel: w326 -> [w344 w351]
                    tunnel: w325 -> [w343 _]
                    frame False {
                      n71 = Format Into String(format string="This ROI was not defined for %s!" ("message"), error in=w347, w343) -> (resulting string=w349:string, error out=w346:errorcluster)  [unwired: 1 in]
                    }
                    frame True {
                      n72 = Unbundle By Name(w352) -> ("ROI Descriptor"=w353:T2)
                      n73 = property class="ImageControl"(reference=w366, error in=w365, "ROI"=w353) -> (error out=w362:errorcluster)  [unwired: 1 out]
                      n74 = Format Into String(format string=" ROI loaded from %s", initial string=w355, w363) -> (resulting string=w358:string)  [unwired: 1 in, 1 out]
                      n75 = case shown="No Error" w362 {
                        tunnel: w361 -> [w373 w377]
                        tunnel: [w371 w377] -> w360
                        tunnel: [w372 "ROI not loaded!" ("t")] -> w359
                        tunnel: w358 -> [w372 _]
                        tunnel: w357 -> [_ w375]
                        tunnel: [w369 w375] -> w356
                        tunnel: [1 ("value") w374] -> w354
                        tunnel: w352 -> [w367 _]
                        tunnel: w351 -> [_ w374]
                        frame No Error {
                          n76 = Build Array (concatenate)(w373, w367) -> (w371:T1[])
                          n77 = Array Size(array=w371) -> (size(s)=w370:i32)
                          n78 = Decrement(x=w370) -> (x-1=w369:i32)
                        }
                        frame Error {
                        }
                      }
                    }
                  }
                }
                frame Error {
                }
              }
            }
            frame "Multiple ROIs v2" {
              w392 = T10 {"Image Control Label"="", "Named ROI Descriptions"=[]}  # Image Control Multiple ROIs Description v2
              # "using default LV XML Read VI modifed by me"
              n79 = Unflatten From XML(xml string=w399, type=w392) -> (value=w391:T10, error out=w390:errorcluster)  [unwired: 1 in]
              n80 = case shown="No Error" w390 {
                selector: w390 -> [w414 w462]
                tunnel: w391 -> [w421 _]
                tunnel: w402 -> [_ w464]
                tunnel: w398 -> [w419 w466]
                tunnel: [w418 w466] -> w397
                tunnel: [w417 w462] -> w388
                tunnel: w400 -> [w416 _]
                tunnel: w401 -> [w415 _]
                tunnel: w396 -> [w412 w465]
                tunnel: [w411 w465] -> w395
                tunnel: [w410 w464] -> w394
                tunnel: [w409 w461] -> w393
                tunnel: [ROI_XML_Format."Exit" ROI_XML_Format."Single ROI v3"] -> w389
                tunnel: [w405 w460] -> w387
                tunnel: w386 -> [w404 w461]
                tunnel: w385 -> [_ w460]
                tunnel: w384 -> [w403 _]
                frame No Error {
                  n81 = Unbundle By Name(w421) -> ("Image Control Label"=w406:string, "Named ROI Descriptions"=w413:T1[])
                  n82 = Equal?(x=w406, y="Phasor Plot Image") -> (x = y?=w405:bool)
                  n83 = Equal?(x=w403, y=w406) -> (x = y?=w420:bool)
                  n84 = case shown="True" w420 {
                    tunnel: w415 -> [_ w448]
                    tunnel: w414 -> [w426 w447]
                    tunnel: [w428 w441] -> w410
                    tunnel: w416 -> [_ w432]
                    tunnel: w403 -> [w424 w446]
                    tunnel: w419 -> [w427 w443]
                    tunnel: [w427 w442] -> w418
                    tunnel: [w425 w444] -> w417
                    tunnel: w413 -> [_ w438]
                    tunnel: w412 -> [w423 w436]
                    tunnel: [w423 w435] -> w411
                    tunnel: [w422 w433] -> w409
                    tunnel: w404 -> [w422 w430]
                    frame False {
                      n85 = Format Into String(format string="This ROI was not defined for %s!" ("message"), error in=w426, w424) -> (resulting string=w428:string, error out=w425:errorcluster)  [unwired: 1 in]
                    }
                    frame True {
                      # "Only shows the last ROI"
                      n86 = Array Size(array=w438) -> (size(s)=w434:i32)
                      n87 = Decrement(x=w434) -> (x-1=w437:i32)
                      n88 = Index Array(array=w438, index=w437) -> (element=w439:T1)
                      n89 = Unbundle By Name(w439) -> ("ROI Descriptor"=w431:T2)
                      n90 = property class="ImageControl"(reference=w448, error in=w447, "ROI"=w431) -> (error out=w444:errorcluster)  [unwired: 1 out]
                      n91 = Format Into String(format string=" ROI loaded from %s", initial string=w446, w432) -> (resulting string=w440:string)  [unwired: 1 in, 1 out]
                      n92 = case shown="Error" w444 {
                        tunnel: w443 -> [w455 w459]
                        tunnel: [w453 w459] -> w442
                        tunnel: [w454 "ROI not loaded!" ("t")] -> w441
                        tunnel: w440 -> [w454 _]
                        tunnel: w438 -> [w449 _]
                        tunnel: w436 -> [_ w457]
                        tunnel: [w451 w457] -> w435
                        tunnel: w434 -> [w450 _]
                        tunnel: [w450 w456] -> w433
                        tunnel: w430 -> [_ w456]
                        frame No Error {
                          n93 = Build Array (concatenate)(w455, w449) -> (w453:T1[])
                          n94 = Array Size(array=w453) -> (size(s)=w452:i32)
                          n95 = Decrement(x=w452) -> (x-1=w451:i32)
                        }
                        frame Error {
                        }
                      }
                    }
                  }
                }
                frame Error {
                }
              }
            }
            frame "Single ROI v3" {
              w468 = T9 {"Image Control Label"="", "Named ROI Description"={"ROI Descriptor"={"Global Rectangle"=[], "Contours"=[]}, "ROI Name"="", "Overlay Color"=0}}  # Single ROI Description v2
              # "using JDP Science JSON Read VI"
              n96 = disable-structure shown="Enabled" {
                disable-tunnel: w477 -> [w494 w504]
                disable-tunnel: [w493 w500] -> w476
                disable-tunnel: [w491 w496] -> w475
                disable-tunnel: [w489 w498] -> w474
                disable-tunnel: w468 -> [w488 w497]
                disable-tunnel: [_ w495] -> w467
                frame Disabled {
                  n97 = call <vilib>:"Easy Read XML File__JKI EasyXML.vi"("LabVIEW Data (Type)"=w488, "XML File Path"=w494) -> ("error out"=w490:errorcluster, "LabVIEW Data"=w492:variant, "XML File Path (duplicate)"=w493:path)  [unwired: 7 in]
                  n98 = Variant To Data(error in=w490, type=w488, Variant=w492) -> (data=w491:T9, error out=w489:errorcluster)
                }
                frame Enabled {
                  n99 = Read from Text File(file (use dialog)=w504, count=-1) -> (refnum out=w501:refnum<file>, text=w502:string, error out=w499:errorcluster)  [unwired: 2 in, 1 out]
                  n100 = call "From JSON Text.vim"("Data Type and Default Value"=w497, "error in (no error)"=w499, "JSON"=w502) -> ("error out"=w498:errorcluster, "Data out"=w496:T9)  [unwired: 7 in]
                  n101 = Close File(refnum=w501, error in=w499) -> (path=w500:path)  [unwired: 1 out]
                  n102 = Not Equal?(x=w497, y=w496) -> (x != y?=w495:bool)
                }
              }
              n103 = case shown="True" w467 {
                tunnel: w475 -> [_ w537]
                tunnel: w470 -> [w511 w521]
                tunnel: w487 -> [_ w536]
                tunnel: w476 -> [_ w535]
                tunnel: w486 -> [w510 w534]
                tunnel: [w510 w533] -> w485
                tunnel: [w505 w532] -> w478
                tunnel: w484 -> [w509 w531]
                tunnel: [w509 w530] -> w483
                tunnel: [w506 w516] -> w482
                tunnel: [w511 w529] -> w481
                tunnel: [w507 w528] -> w480
                tunnel: [ROI_XML_Format."Multiple ROIs v3" w522] -> w479
                tunnel: w473 -> [w507 w524]
                tunnel: w472 -> [w506 _]
                tunnel: w471 -> [_ w520]
                tunnel: [w505 w519] -> w469
                tunnel: w474 -> [_ w525]
                frame False {
                  n104 = xnode "Error Ring"() -> ("error out"=w505:errorcluster)
                }
                frame True {
                  n105 = Unbundle By Name(w537) -> ("Image Control Label"=w518:string, "Named ROI Description.ROI Name"=w523:string, "Named ROI Description"=w526:T1)
                  n106 = Equal?(x=w520, y=w518) -> (x = y?=w527:bool)
                  n107 = Equal?(x=w518, y="Phasor Plot Image") -> (x = y?=w516:bool)
                  n108 = case shown="True" w527 {
                    tunnel: w526 -> [_ w557]
                    tunnel: w536 -> [_ w568]
                    tunnel: [w545 w563] -> w529
                    tunnel: w535 -> [_ w567]
                    tunnel: w518 -> [_ w560]
                    tunnel: w521 -> [_ w548]
                    tunnel: w534 -> [w544 w565]
                    tunnel: [w544 w564] -> w533
                    tunnel: [w538 w566] -> w532
                    tunnel: w531 -> [w543 w562]
                    tunnel: [w543 w561] -> w530
                    tunnel: [w541 w559] -> w528
                    tunnel: w525 -> [w542 w556]
                    tunnel: w524 -> [w541 w555]
                    tunnel: w523 -> [_ w554]
                    tunnel: [ROI_XML_Format."Multiple ROIs v3" w549] -> w522
                    tunnel: w520 -> [w539 _]
                    tunnel: [w538 w547] -> w519
                    frame False {
                      n109 = Format Into String(format string="This ROI was not defined for %s!" ("message"), error in=w542, w539) -> (resulting string=w545:string, error out=w538:errorcluster)  [unwired: 1 in]
                    }
                    frame True {
                      n110 = Unbundle By Name(w557) -> ("ROI Descriptor"=w558:T2, "ROI Descriptor.Global Rectangle"=w553:i32[])
                      n111 = Empty String/Path?(string/path=w554) -> (empty?=w551:bool)
                      n112 = Empty Array?(array=w553) -> (empty?=w552:bool)
                      n113 = Or(x=w552, y=w551) -> (x .or. y?=w550:bool)
                      n114 = case shown="True" w550 {
                        tunnel: w568 -> [w585 _]
                        tunnel: w567 -> [w583 _]
                        tunnel: [w582 w599] -> w566
                        tunnel: w565 -> [w581 w601]
                        tunnel: [w580 w601] -> w564
                        tunnel: [w579 w598] -> w563
                        tunnel: w562 -> [w577 w602]
                        tunnel: [w576 w602] -> w561
                        tunnel: w560 -> [w569 _]
                        tunnel: [w575 w600] -> w559
                        tunnel: w558 -> [w574 _]
                        tunnel: w557 -> [w573 _]
                        tunnel: w556 -> [w570 w599]
                        tunnel: w555 -> [w572 w600]
                        tunnel: [ROI_XML_Format."Exit" ROI_XML_Format."Multiple ROIs v3"] -> w549
                        tunnel: w548 -> [_ w598]
                        tunnel: [w570 w597] -> w547
                        frame False {
                          n115 = property class="ImageControl"(reference=w585, error in=w570, "ROI"=w574) -> (error out=w582:errorcluster)  [unwired: 1 out]
                          n116 = Format Into String(format string=" ROI loaded from %s", initial string=w569, w583) -> (resulting string=w578:string)  [unwired: 1 in, 1 out]
                          n117 = case shown="No Error" w582 {
                            tunnel: w581 -> [w592 w596]
                            tunnel: [w590 w596] -> w580
                            tunnel: [w591 "ROI not loaded!" ("t")] -> w579
                            tunnel: w578 -> [w591 _]
                            tunnel: w577 -> [_ w594]
                            tunnel: [w588 w594] -> w576
                            tunnel: [1 ("value") w593] -> w575
                            tunnel: w573 -> [w586 _]
                            tunnel: w572 -> [_ w593]
                            frame No Error {
                              n118 = Build Array (concatenate)(w592, w586) -> (w590:T1[])
                              n119 = Array Size(array=w590) -> (size(s)=w589:i32)
                              n120 = Decrement(x=w589) -> (x-1=w588:i32)
                            }
                            frame Error {
                            }
                          }
                        }
                        frame True {
                          # "Not a valid single ROI file: try multiple ROI decoding"
                          n121 = xnode "Error Ring"() -> ("error out"=w597:errorcluster)
                        }
                      }
                    }
                  }
                }
              }
            }
            frame "Multiple ROIs v3" {
              w610 = T10 {"Image Control Label"="", "Named ROI Descriptions"=[]}  # Image Control Multiple ROIs Description v2
              # "using JDP Science JSON Read VI"
              n122 = disable-structure shown="Enabled" {
                disable-tunnel: w617 -> [w634 w641]
                disable-tunnel: [w633 w638] -> w616
                disable-tunnel: [w630 w636] -> w615
                disable-tunnel: [w629 w640] -> w614
                disable-tunnel: w610 -> [w628 w637]
                disable-tunnel: [_ w635] -> w609
                frame Disabled {
                  n123 = call <vilib>:"Easy Read XML File__JKI EasyXML.vi"("LabVIEW Data (Type)"=w628, "XML File Path"=w634) -> ("error out"=w631:errorcluster, "LabVIEW Data"=w632:variant, "XML File Path (duplicate)"=w633:path)  [unwired: 7 in]
                  n124 = Variant To Data(error in=w631, type=w628, Variant=w632) -> (data=w630:T10, error out=w629:errorcluster)
                }
                frame Enabled {
                  n125 = Read from Text File(file (use dialog)=w641, count=-1) -> (refnum out=w639:refnum<file>, text=w643:string, error out=w642:errorcluster)  [unwired: 2 in, 1 out]
                  n126 = call "From JSON Text.vim"("Data Type and Default Value"=w637, "error in (no error)"=w642, "JSON"=w643) -> ("error out"=w640:errorcluster, "Data out"=w636:T10)  [unwired: 7 in]
                  n127 = Close File(refnum=w639, error in=w642) -> (path=w638:path)  [unwired: 1 out]
                  n128 = Not Equal?(x=w637, y=w636) -> (x != y?=w635:bool)
                }
              }
              n129 = case shown="True" w609 {
                tunnel: w615 -> [_ w677]
                tunnel: w627 -> [_ w658]
                tunnel: w625 -> [w653 w675]
                tunnel: [w653 w674] -> w624
                tunnel: [w645 w673] -> w608
                tunnel: w616 -> [w648 w672]
                tunnel: w626 -> [_ w671]
                tunnel: w623 -> [w652 w668]
                tunnel: [w652 w667] -> w622
                tunnel: [w647 w666] -> w621
                tunnel: [w650 w665] -> w620
                tunnel: [ROI_XML_Format."Exit" ROI_XML_Format."Exit"] -> w619
                tunnel: [w646 w661] -> w618
                tunnel: w613 -> [w650 w660]
                tunnel: w612 -> [w646 _]
                tunnel: w611 -> [_ w659]
                tunnel: w614 -> [_ w670]
                frame False {
                  n130 = Format Into String(format string="Could not load ROI(s) in %s!" ("message"), w648) -> (resulting string=w647:string)  [unwired: 2 in, 1 out]
                  n131 = xnode "Error Ring"() -> ("error out"=w645:errorcluster)
                }
                frame True {
                  n132 = Unbundle By Name(w677) -> ("Image Control Label"=w662:string, "Named ROI Descriptions"=w669:T1[])
                  n133 = Equal?(x=w659, y=w662) -> (x = y?=w676:bool)
                  n134 = Equal?(x=w662, y="Phasor Plot Image") -> (x = y?=w661:bool)
                  n135 = case shown="True" w676 {
                    tunnel: w671 -> [_ w704]
                    tunnel: w670 -> [w682 w703]
                    tunnel: [w684 w698] -> w666
                    tunnel: w672 -> [_ w688]
                    tunnel: w659 -> [w680 w687]
                    tunnel: w675 -> [w683 w700]
                    tunnel: [w683 w699] -> w674
                    tunnel: [w681 w701] -> w673
                    tunnel: w669 -> [_ w695]
                    tunnel: w668 -> [w679 w693]
                    tunnel: [w679 w692] -> w667
                    tunnel: [w678 w691] -> w665
                    tunnel: w660 -> [w678 w689]
                    tunnel: w658 -> [_ _]
                    frame False {
                      n136 = Format Into String(format string="This ROI was not defined for %s!" ("message"), error in=w682, w680) -> (resulting string=w684:string, error out=w681:errorcluster)  [unwired: 1 in]
                    }
                    frame True {
                      # "Only shows the last ROI"
                      n137 = Array Size(array=w695) -> (size(s)=w686:i32)
                      n138 = Decrement(x=w686) -> (x-1=w694:i32)
                      n139 = Index Array(array=w695, index=w694) -> (element=w696:T1)
                      n140 = Unbundle By Name(w696) -> ("ROI Descriptor"=w690:T2)
                      n141 = property class="ImageControl"(reference=w704, error in=w703, "ROI"=w690) -> (error out=w701:errorcluster)  [unwired: 1 out]
                      n142 = Format Into String(format string="%d %s ROIs loaded from %s", w686, w687, w688) -> (resulting string=w697:string)  [unwired: 2 in, 1 out]
                      n143 = case shown="No Error" w701 {
                        tunnel: w700 -> [w711 w715]
                        tunnel: [w709 w715] -> w699
                        tunnel: [w710 "ROI not loaded!" ("t")] -> w698
                        tunnel: w697 -> [w710 _]
                        tunnel: w695 -> [w705 _]
                        tunnel: w693 -> [_ w713]
                        tunnel: [w707 w713] -> w692
                        tunnel: w686 -> [w706 _]
                        tunnel: [w706 w712] -> w691
                        tunnel: w689 -> [_ w712]
                        frame No Error {
                          n144 = Build Array (concatenate)(w711, w705) -> (w709:T1[])
                          n145 = Array Size(array=w709) -> (size(s)=w708:i32)
                          n146 = Decrement(x=w708) -> (x-1=w707:i32)
                        }
                        frame Error {
                        }
                      }
                    }
                  }
                }
              }
            }
            frame "Exit" {
              # "Move on to next file"
              n147 = xnode "Error Ring"() -> ("error out"=w717:errorcluster)
              n148 = Select(t=w718, s=w720, f=w717) -> (s? t:f=w719:errorcluster)
            }
          }
        }
        n149 = Concatenate Strings(w98, w100, "\n" ("string")) -> (w99:string)
        n150 = Compound Arithmetic op=ADD(w96, w95) -> (w97:i32)
      }
      n151 = call "High Resolution Timing.vi"("relative seconds (NaN)"=w71, "Error In"=w82) -> ("elapsed (relative) seconds"=w70:dbl, "Error Out"=w72:errorcluster)  [unwired: 15 in, 1 out]
    }
    frame True {
    }
  }
  "Updated ROIs" <- w9
  "Current ROI" <- w10
  "Phasor Plot Image" <- w17
  "# ROIs Loaded" <- w14
  "Time (s)" <- w6
  "Message" <- w2
  n152 = case shown="\"Phasor Plot Image\"" w8 {
    tunnel: w10 -> [w738 w751]
    tunnel: w9 -> [w737 w750]
    tunnel: w1 -> [w733 w746]
    tunnel: [w730 w744] -> w7
    frame "Source Image", Default {
      n153 = call "Alligator Variables Storage.vi"("Get(F)/Set"=TRUE, "AlliGator Variable"=AlliGator_Variables_List."Source Image:ROIs" ("Alligator Variable"), "Error In"=w733, "Data in"=w737) -> ("Error Out"=w736:errorcluster)  [unwired: 5 in, 2 out]
      n154 = call "Alligator Variables Storage.vi"("Get(F)/Set"=TRUE, "AlliGator Variable"=AlliGator_Variables_List."Source Image:Current ROI" ("Alligator Variable"), "Error In"=w733, "Data in"=w738) -> ("Error Out"=w735:errorcluster)  [unwired: 5 in, 2 out]
      n155 = Merge Errors(w735, w736) -> (w731:errorcluster)
      n156 = call "AlliGator Get Source Image ROI Event Refnum.vi"() -> ("Source Image ROI Event Refnum"=w734:T12)
      n157 = Generate User Event(user event=w734, event data cluster=AlliGator_ROI_Manager_Actions."Update ROI Manager Window" ("event data"), error in=w731) -> (error out=w730:errorcluster)  [unwired: 1 in, 1 out]
    }
    frame "Phasor Plot Image" {
      n158 = call "Alligator Variables Storage.vi"("Get(F)/Set"=TRUE, "AlliGator Variable"=AlliGator_Variables_List."Phasor Plot:ROIs" ("Alligator Variable"), "Error In"=w746, "Data in"=w750) -> ("Error Out"=w749:errorcluster)  [unwired: 5 in, 2 out]
      n159 = call "Alligator Variables Storage.vi"("Get(F)/Set"=TRUE, "AlliGator Variable"=AlliGator_Variables_List."Phasor Plot:Current ROI" ("Alligator Variable"), "Error In"=w746, "Data in"=w751) -> ("Error Out"=w748:errorcluster)  [unwired: 5 in, 2 out]
      n160 = Merge Errors(w748, w749) -> (w745:errorcluster)
      n161 = call "AlliGator Get Phasor Plot ROI Event Refnum.vi"() -> ("Phasor Plot ROI Event Refnum"=w747:T12)
      n162 = Generate User Event(user event=w747, event data cluster=AlliGator_ROI_Manager_Actions."Update ROI Manager Window" ("event data"), error in=w745) -> (error out=w744:errorcluster)  [unwired: 1 in, 1 out]
    }
  }
  "Error Out" <- w7
